vi "Get-action.vi"(8 "error in (no error)":errorcluster, 9 "Position in":i32, 11 "Sequence in":refnum<class "Action-sequence.lvclass">) -> (0 "error out":errorcluster, 1 "Position":i32, 2 "Action":refnum<class "Action.lvclass">, 3 "Sequence out":refnum<class "Action-sequence.lvclass">)   [LabVIEW 2013, in "PowderDeposition.lvlib" / "Action-sequence.lvclass"]
uses:
  Action-sequence.lvclass
  Action/Action.lvclass
  Action-sequence.lvclass/Action-sequence.ctl
  Main/Custom-errors.ctl
  Main/PD-Main.lvclass
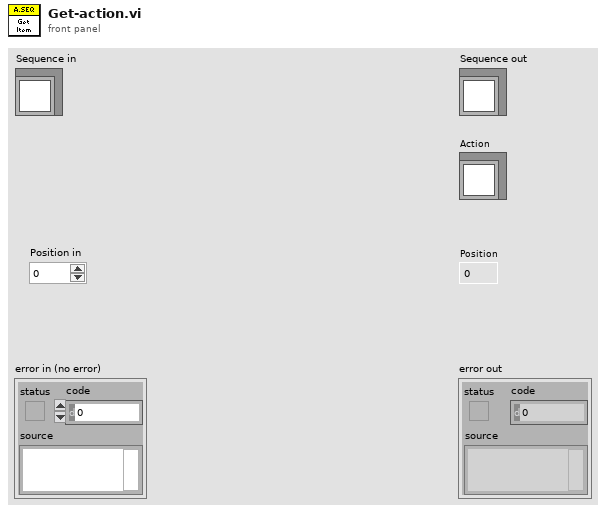
[diagram p1: front panel]
types:
  T1 = typedef "PowderDeposition.lvlib/PD-Main.lvclass/Custom-errors.ctl" = enum16{"Not implemented", "Command not recognized", "Invalid input", "Timeout", "Load file failed", "Action failed", "Action invalid", "Motor inactive", "Not in range", "Unsafe state"}
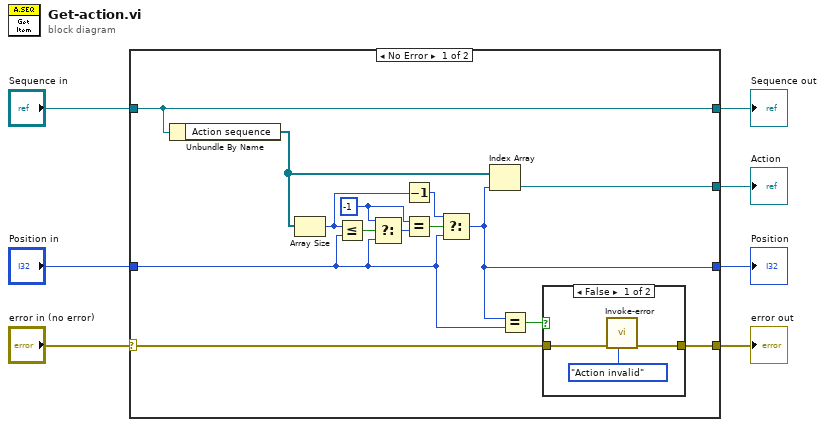
[diagram p0: block diagram]
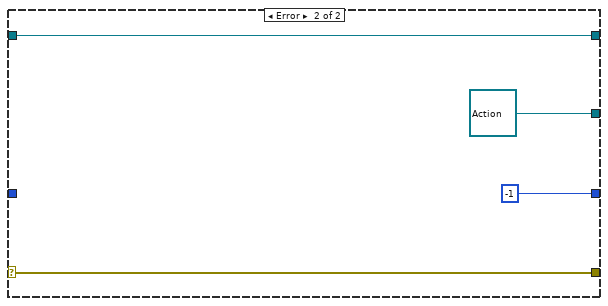
[diagram p3: hidden frame]
diagram:
  n1 = case shown="No Error" "error in (no error)" {
    selector: "error in (no error)" -> [w12 w29]
    tunnel: [w11 w29] -> w6
    tunnel: [w21 w28] -> w4
    tunnel: "Sequence in" -> [w21 w28]
    tunnel: "Position in" -> [w8 _]
    tunnel: [w9 -1 ("Position")] -> w2
    tunnel: [w13 refnum<class "Action.lvclass"> refnum ("Action.lvclass")] -> w1
    frame No Error {
      w18 = -1 ("t")
      n2 = Unbundle By Name(w21) -> ("Action sequence"=w14:refnum<class "Action.lvclass">[])
      n3 = Array Size(array=w14) -> (size(s)=w16:i32)
      n4 = Less Or Equal?(x=w16, y=w8) -> (x <= y?=w20:bool)
      n5 = Select(t=w18, s=w20, f=w8) -> (s? t:f=w19:i32)
      n6 = Decrement(x=w16) -> (x-1=w15:i32)
      n7 = Equal?(x=w18, y=w19) -> (x = y?=w17:bool)
      n8 = Select(t=w15, s=w17, f=w8) -> (s? t:f=w9:i32)
      n9 = Index Array(array=w14, index=w9) -> (element=w13:refnum<class "Action.lvclass">)
      n10 = Equal?(x=w9, y=w8) -> (x = y?=w10:bool)
      n11 = case shown="False" w10 {
        tunnel: w12 -> [w24 w25]
        tunnel: [w23 w25] -> w11
        frame False {
          n12 = call "Invoke-error.vi"("Error"=Custom-errors."Action invalid", "error in (no error)"=w24) -> ("error out"=w23:errorcluster)  [unwired: 9 in]
        }
        frame True {
        }
      }
    }
    frame Error {
    }
  }
  "error out" <- w6
  "Sequence out" <- w4
  "Position" <- w2
  "Action" <- w1
